vi "DV Prototype Global Variables.vi"() -> ()   [LabVIEW 2014]
uses:
  <vilib>/Utility/miscctls.llb/LVRectTypeDef.ctl
  <vilib>/Utility/miscctls.llb/LVPointTypeDef.ctl
panel:
  out "Server IP":string
  in  "System Tray":enum16{"Enabled", "Disabled"}(ring)
  in  "Active Display":u16
  out "Pane Origin":T1[](array[typedef])
  in  "FP Size":cluster{"Width":i16, "Height":i16}={"Width"=1711, "Height"=1001}
  in  "FP Bounds":T2={"Left"=105, "Top"=-7, "Right"=1816, "Bottom"=994}
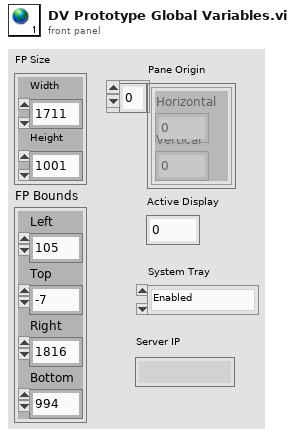
[diagram p1: front panel]
types:
  T1 = typedef "LVPointTypeDef.ctl" = cluster{"Horizontal":i16, "Vertical":i16}
  T2 = typedef "LVRectTypeDef.ctl" = cluster{"Left":i16, "Top":i16, "Right":i16, "Bottom":i16}
diagram:
